vi "PickRobots.vi"(0 "object in":refnum<class "StandardAttackPlay.lvclass">, 2 "GameRef":refnum<data-value>, 5 "error in (no error)":errorcluster) -> (14 "object out":refnum<class "StandardAttackPlay.lvclass">, 16 "Robots":refnum<class "Robot.lvclass">[](array[class]), 19 "error out":errorcluster)   [LabVIEW 2023, in "StandardAttackPlay.lvclass"]
uses:
  StandardAttackPlay.lvclass
  C:/Users/ebert/Documents/codes/SSL/repo/SSL_AI/NewSTP/NewPlays/Play_v2_class/Play_v2.lvclass
  Robot_class/Robot.lvclass
  Game_class/Game.lvclass
  Game_class/Game.lvclass/Game.ctl
  Team_class/Team.lvclass/Team.ctl
  Object_class/Object.lvclass/Object.ctl
  Zone_class/Zone.lvclass
  Zone_class/zones.ctl
  Robot_class/roles.ctl
  SupportAttackerRole/SupportAttackerRole.lvclass
  C:/Users/ebert/Documents/codes/SSL/repo/SSL_AI/NewSTP/NewRoles/Role_v2_class/Role_v2.lvclass
  Robot_class/Robot.lvclass/Robot.ctl
  Robot_class/Write role.vi
  Game_class/Read AllyRef.vi
  Game_class/Read BallRef.vi
  Game_class/Read FieldRef.vi
  Object_class/Read position(x,y).vi
  Team_class/Read RobotRef.vi
  Ball_class/Ball.lvclass
  C:/Users/ebert/Documents/codes/SSL/repo/SSL_AI/Object_class/Object.lvclass
  Ally_class/Ally.lvclass
  C:/Users/ebert/Documents/codes/SSL/repo/SSL_AI/Team_class/Team.lvclass
  Field_class/Field.lvclass
  NewRoles/Role_v2_class/Role_v2.lvclass
  Play_v2_class/Play_v2.lvclass
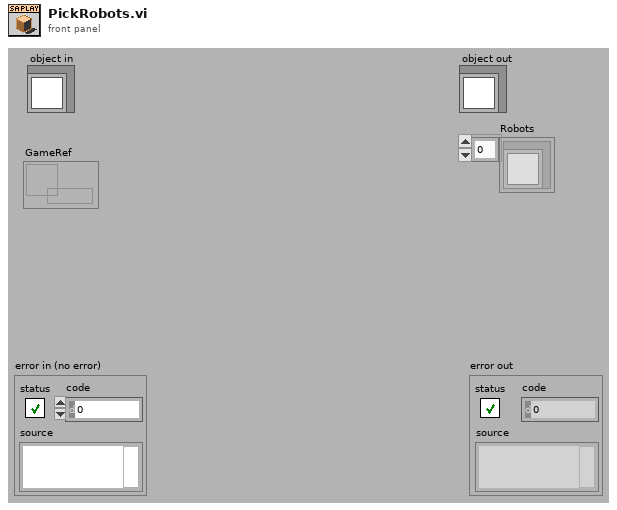
[diagram p1: front panel]
types:
  T1 = typedef "STPParameters.ctl" = cluster{"Skills":T2, "TestSkill":T4, "Events":cluster{"distanceToBallPossession":dbl, "timeForPossessionThreshold":dbl}, "Criteria":cluster{"OpenAngleToGoal":cluster{"minAngle":dbl, "maxAngle":dbl, "minEvaluation":dbl}, "PassDistance":cluster{"maxDistance":dbl, "minDistance":dbl}, "ShotInterception":cluster{"shotSpeed":dbl, "minEnemySpeed":dbl, "minEvaluation":dbl, "maxEnemySpeed":dbl}, "OneTouchShot":cluster{"MaxAngle":dbl, "minEvaluation":dbl}, "PassInterception":cluster{"minEnemySpeed":dbl, "maxEnemySpeed":dbl, "chipPassDistance":dbl, "chipPassEval":dbl, "minEvaluation":dbl}}, "minPassSpeed":dbl, "maxPassSpeed":dbl, "AllyTeamIds":T5[], "ReceiverSpeed":dbl, "minEvaluationToShoot":dbl}
  T2 = typedef "Skills.ctl" = cluster{"CirculateBall":T3, "ProtectBall":cluster{"DistanceFromBall":dbl}}
  T3 = typedef "CIrculateSkillParameters.ctl" = cluster{"rotationAngle":dbl, "velocityFactor":dbl, "OrientationFactor":dbl}
  T4 = typedef "TestSkills.ctl" = enum16{"AlignSkill", "PassSkill", "CirculateBall", "OneTouchShotSkill", "KickToSkill_v2", "ShootSkill", "InterceptBall", "Exit", "GoToSkill_v2"}
  T5 = typedef "AllyTeam.ctl" = enum16{"Keeper", "Defender", "Attacker"}
  T6 = typedef "Zone.lvclass/zones.ctl" = enum16{"leftMidField", "rightMidField", "MidField", "leftWing", "rightWing", "LeftSide", "RightSide", "Field", "Size"}
  T7 = typedef "roles.ctl" = enum16{"SimpleBallPlacement", "BallPlacementAllyPasser", "BallPlacementAllyReceiver", "BallPlacementEnemy", "5Robots5th", "PassBestReceiver", "5Robots4th", "5Robots3rd", "5Robots2nd", "5Robots1st", "PassBestRobot", "WaitPass", "ABCThirdKicker", "ABCFirstKicker", "ABCSecondKicker", "Tabler", "TableFinalizer", "PrepareRollToPassRoller", "PrepareRollToPassReceiver", "SimplePassRoll", "SimplePassRollReceiver", "PenaltyDefense", "PreparePassReceiver 2", "PreparePassReceiver 1", "PassObserver", "Timeout", "Goto", "ZigZag", "None", "BallOutOfField", "DefenderArea", "Duelist", "AttackerStop", "FollowAttacker", "KeeperRole", "KickPenalty", "AttackerAimGoal", "AttackerBlock", "Marker", "Halt", "Shoot", "PassKicker", "PassReceiver", "TestRole", "PenaltyAttacker", "PrimaryAttackerRole", "SupportAttackerRole"}
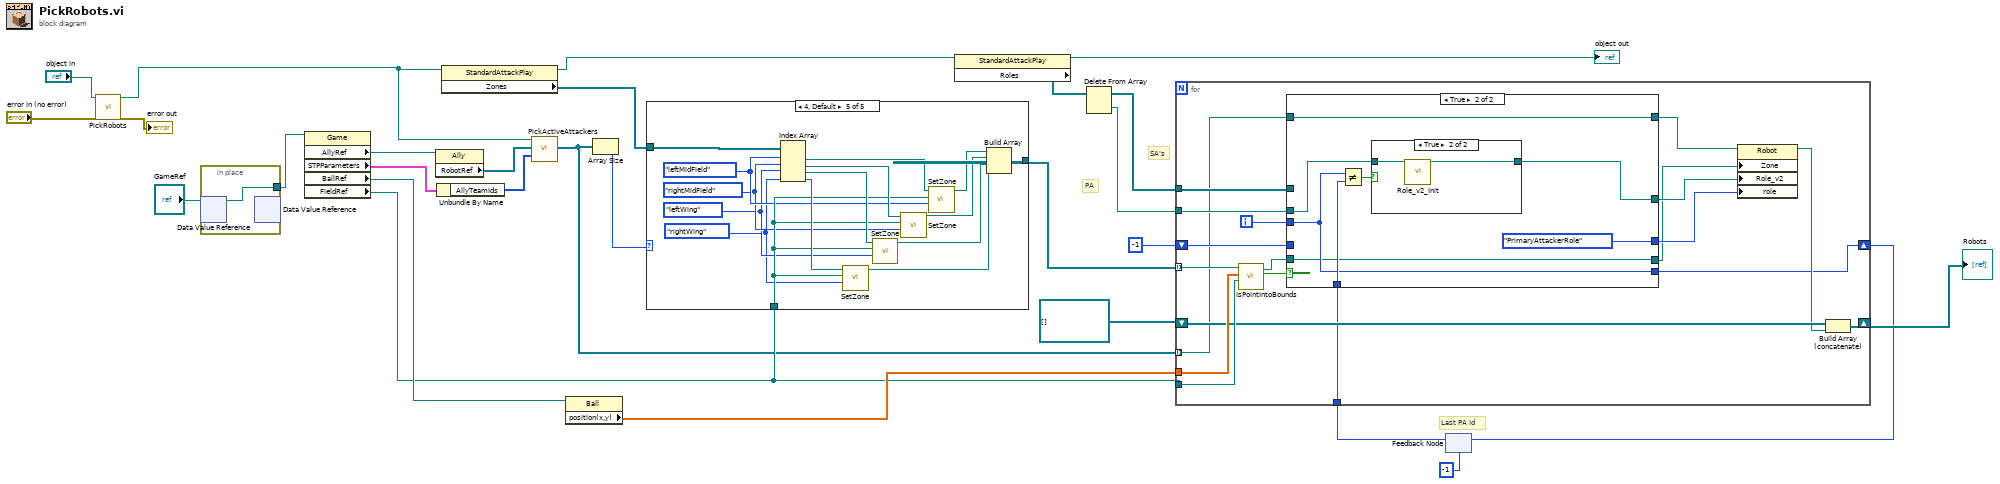
[diagram p0: block diagram]
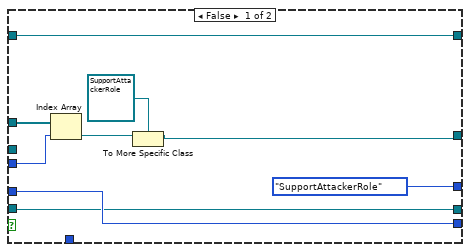
[diagram p2: hidden frame]
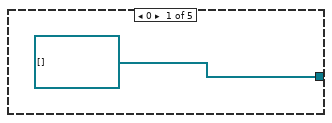
[diagram p4: hidden frame]
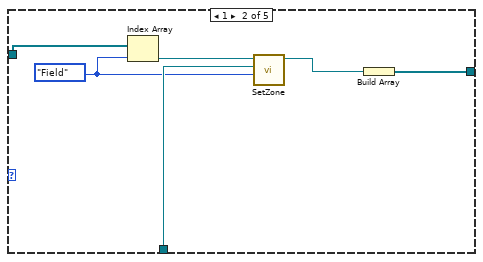
[diagram p5: hidden frame]
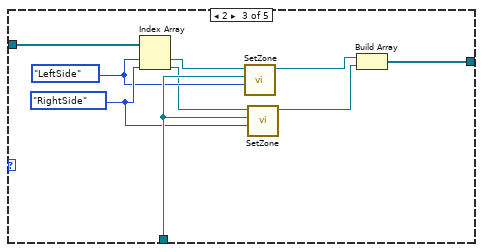
[diagram p6: hidden frame]
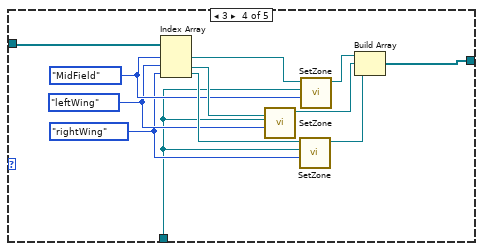
[diagram p7: hidden frame]
diagram:
  # "SA's"
  # "PA"
  # "Last PA Id"
  n1 = call-parent "PickRobots.vi"("object in"="object in", "error in (no error)"="error in (no error)") -> ("object out"=w4:refnum<class "StandardAttackPlay.lvclass">, "error out"=→"error out":errorcluster)  [unwired: 15 in, 1 out]
  n2 = in-place {
    in-place-border: [w29] -> w12
    n3 = in-place-dvr #1("GameRef") -> (w29:refnum<class "Game.lvclass">)  [unwired: 1 out]
    n4 = in-place-dvr #1() -> ()  [unwired: 1 in, 2 out]
  }
  n5 = property class="Game"(reference=w12) -> ("AllyRef"=w25:refnum<class "Ally.lvclass">, "STPParameters"=w24:T1, "BallRef"=w22:refnum<class "Ball.lvclass">, "FieldRef"=w15:refnum<class "Field.lvclass">)  [unwired: 1 in, 2 out]
  n6 = property class="Ally"(reference=w25) -> ("RobotRef"=w3:refnum<class "Robot.lvclass">[])  [unwired: 1 in, 2 out]
  n7 = Unbundle By Name(w24) -> ("AllyTeamIds"=w2:T5[])
  n8 = property class="StandardAttackPlay"(reference=w4) -> (reference out=w17:refnum<class "StandardAttackPlay.lvclass">, "Zones"=w19:refnum<class "Zone.lvclass">[])  [unwired: 1 in, 1 out]
  n9 = call-dynamic "PickActiveAttackers.vi"("object in"=w4, "AllyRobots"=w3, "AllyTeamIds"=w2) -> ("ActiveAttackers"=w1:refnum<class "Robot.lvclass">[])  [unwired: 14 in, 2 out]
  n10 = property class="Ball"(reference=w22) -> ("position(x,y)"=w21:dbl[])  [unwired: 1 in, 2 out]
  n11 = Array Size(array=w1) -> (size(s)=w23:i32)
  n12 = case shown="4, Default" w23 {
    tunnel: [refnum<class "Zone.lvclass">[] [] ("Zones") w35 w37 w56 w71] -> w20
    tunnel: w19 -> [_ w36 w45 w57 w72]
    tunnel: w15 -> [_ w32 w44 w49 w66]
    frame 0 {
    }
    frame 1 {
      w31 = zones."Field" ("Enum")
      n13 = Index Array(array=w36, index=w31) -> (element=w34:refnum<class "Zone.lvclass">)
      n14 = call-dynamic "SetZone.vi"("Enum"=w31, "Field"=w32, "object in"=w34) -> ("object out"=w33:refnum<class "Zone.lvclass">)  [unwired: 7 in, 1 out]
      n15 = Build Array(w33) -> (w35:refnum<class "Zone.lvclass">[])
    }
    frame 2 {
      w43 = zones."RightSide" ("Enum")
      w42 = zones."LeftSide" ("Enum")
      n16 = Index Array(array=w45, index #1=w42, index #2=w43) -> (element #1=w41:refnum<class "Zone.lvclass">, element #2=w40:refnum<class "Zone.lvclass">)
      n17 = call-dynamic "SetZone.vi"("Enum"=w42, "Field"=w44, "object in"=w41) -> ("object out"=w39:refnum<class "Zone.lvclass">)  [unwired: 7 in, 1 out]
      n18 = call-dynamic "SetZone.vi"("Enum"=w43, "Field"=w44, "object in"=w40) -> ("object out"=w38:refnum<class "Zone.lvclass">)  [unwired: 7 in, 1 out]
      n19 = Build Array(w39, w38) -> (w37:refnum<class "Zone.lvclass">[])
    }
    frame 3 {
      w50 = zones."rightWing" ("Enum")
      w51 = zones."leftWing" ("Enum")
      w52 = zones."MidField" ("Enum")
      n20 = Index Array(array=w57, index #1=w52, index #2=w51, index #3=w50) -> (element #1=w55:refnum<class "Zone.lvclass">, element #2=w54:refnum<class "Zone.lvclass">, element #3=w53:refnum<class "Zone.lvclass">)
      n21 = call-dynamic "SetZone.vi"("Enum"=w51, "Field"=w49, "object in"=w54) -> ("object out"=w47:refnum<class "Zone.lvclass">)  [unwired: 7 in, 1 out]
      n22 = call-dynamic "SetZone.vi"("Enum"=w50, "Field"=w49, "object in"=w53) -> ("object out"=w46:refnum<class "Zone.lvclass">)  [unwired: 7 in, 1 out]
      n23 = call-dynamic "SetZone.vi"("Enum"=w52, "Field"=w49, "object in"=w55) -> ("object out"=w48:refnum<class "Zone.lvclass">)  [unwired: 7 in, 1 out]
      n24 = Build Array(w48, w47, w46) -> (w56:refnum<class "Zone.lvclass">[])
    }
    frame 4, Default {
      w64 = zones."rightMidField" ("Enum")
      w62 = zones."rightWing" ("Enum")
      w63 = zones."leftWing" ("Enum")
      w65 = zones."leftMidField" ("Enum")
      n25 = Index Array(array=w72, index #1=w65, index #2=w64, index #3=w63, index #4=w62) -> (element #1=w67:refnum<class "Zone.lvclass">, element #2=w68:refnum<class "Zone.lvclass">, element #3=w69:refnum<class "Zone.lvclass">, element #4=w70:refnum<class "Zone.lvclass">)
      n26 = call-dynamic "SetZone.vi"("Enum"=w62, "Field"=w66, "object in"=w70) -> ("object out"=w60:refnum<class "Zone.lvclass">)  [unwired: 7 in, 1 out]
      n27 = call-dynamic "SetZone.vi"("Enum"=w63, "Field"=w66, "object in"=w69) -> ("object out"=w59:refnum<class "Zone.lvclass">)  [unwired: 7 in, 1 out]
      n28 = call-dynamic "SetZone.vi"("Enum"=w64, "Field"=w66, "object in"=w68) -> ("object out"=w58:refnum<class "Zone.lvclass">)  [unwired: 7 in, 1 out]
      n29 = call-dynamic "SetZone.vi"("Enum"=w65, "Field"=w66, "object in"=w67) -> ("object out"=w61:refnum<class "Zone.lvclass">)  [unwired: 7 in, 1 out]
      n30 = Build Array(w61, w58, w59, w60) -> (w71:refnum<class "Zone.lvclass">[])
    }
  }
  n31 = property class="StandardAttackPlay"(reference=w17) -> (reference out=→"object out":refnum<class "StandardAttackPlay.lvclass">, "Roles"=w7:refnum<class "Role_v2.lvclass">[])  [unwired: 1 in, 1 out]
  n32 = Delete From Array(array=w7) -> (deleted portion=w6:refnum<class "Role_v2.lvclass">, array with subset deleted=w5:refnum<class "Role_v2.lvclass">[])  [unwired: 2 in]
  n33 = feedback #2(-1) -> (w10:i32)
  n34 = for {
    tunnel: w21 -> [w91]
    tunnel: w20 -> [w90] mode=indexing
    tunnel: w1 -> [w76] mode=indexing
    shift-right: [w86] -> w18
    shift-left: refnum<class "Robot.lvclass">[] [] -> [w88]
    tunnel: w15 -> [w89]
    tunnel: w5 -> [w84]
    tunnel: w6 -> [w82]
    tunnel: w10 -> [w80]
    shift-right: [w77] -> w8
    shift-left: -1 -> [w78]
    i -> [w81]
    n35 = call-dynamic "IsPointIntoBounds.vi"("Field"=w89, "Point"=w91, "object in"=w90) -> ("IntoBounds"=w79:bool, "object out"=w74:refnum<class "Zone.lvclass">)  [unwired: 6 in, 1 out]
    n36 = case shown="True" w79 {
      tunnel: [roles."SupportAttackerRole" ("role") roles."PrimaryAttackerRole" ("role")] -> w85
      tunnel: w84 -> [w97 _]
      tunnel: [w92 w101] -> w83
      tunnel: w82 -> [_ w104]
      tunnel: w81 -> [w99 w105]
      tunnel: w80 -> [_ w107]
      tunnel: [w98 w105] -> w77
      tunnel: w78 -> [w98 _]
      tunnel: w76 -> [w93 w103]
      tunnel: [w93 w103] -> w75
      tunnel: w74 -> [w94 w102]
      tunnel: [w94 w102] -> w73
      frame False {
        n37 = Index Array(array=w97, index=w99) -> (element=w95:refnum<class "Role_v2.lvclass">)
        n38 = To More Specific Class(target class=refnum<class "SupportAttackerRole.lvclass"> refnum ("SupportAttackerRole.lvclass"), reference=w95) -> (specific class reference=w92:refnum<class "SupportAttackerRole.lvclass">)  [unwired: 1 in, 1 out]
      }
      frame True {
        n39 = Not Equal?(x=w105, y=w107) -> (x != y?=w106:bool)
        n40 = case shown="True" w106 {
          tunnel: w104 -> [w109 w111]
          tunnel: [w109 w110] -> w101
          frame False {
          }
          frame True {
            n41 = call "Role_v2_Init.vi"("object in"=w111) -> ("object out"=w110:refnum<class "Role_v2.lvclass">)  [unwired: 17 in, 1 out]
          }
        }
      }
    }
    n42 = property class="Robot"(reference=w75, "Zone"=w73, "Role_v2"=w83, "role"=w85) -> (reference out=w87:refnum<class "Robot.lvclass">)  [unwired: 1 in, 1 out]
    n43 = Build Array (concatenate)(w88, w87) -> (w86:refnum<class "Robot.lvclass">[])
  }
  "Robots" <- w18
  n44 = feedback-in #2(w8) -> ()
